vi "Initialize - Set Time Stamp.vi"(8 "error in (no error)":errorcluster, 11 "Device Item Ref in":T1 format="%.0x") -> (0 "error out":errorcluster, 2 "Path":string, 3 "Device Item Ref out":T1 format="%.0x")   [LabVIEW 2019, in "UDP-Custom-Device System Explorer.lvlib"]
doc: "Set the TimeStamp Ref Device Property to the System Time channel."
uses:
  UDP-Custom-Device System Explorer.lvlib
  <vilib>/NI VeriStand/Custom Device API/Custom Device Item Ref.ctl
  <vilib>/NI VeriStand/Custom Device Tools/Custom Device Utility Library/Custom Device Utility Library.lvlib
  <vilib>/NI VeriStand/Custom Device API/Custom Device API.lvlib
  Property Accessors/Main Accessors.lvlib
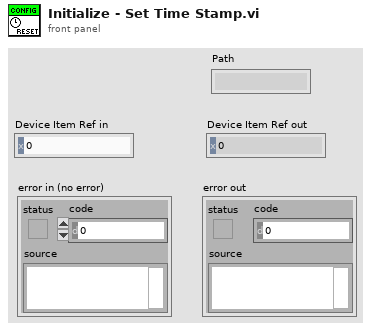
[diagram p1: front panel]
types:
  T1 = typedef "Custom Device API.lvlib/Custom Device Item Ref.ctl" = u64
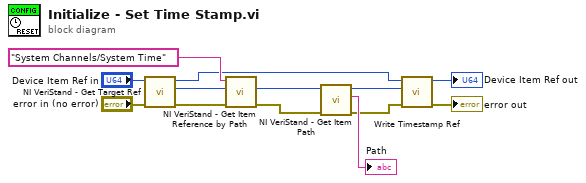
[diagram p0: block diagram]
diagram:
  n1 = call <vilib>:"NI VeriStand - Get Target Ref.vi"("error in"="error in (no error)", "Item Ref in"="Device Item Ref in") -> ("error out"=w12:errorcluster, "Target Ref"=w13:T1, "Item Ref out"=w5:T1)  [unwired: 6 in, 1 out]
  n2 = call <vilib>:"NI VeriStand - Get Item Reference by Path.vi"("error in (no error)"=w12, "Root Ref"=w13, "Item Path in"="System Channels/System Time" ("Relative Item Path")) -> ("error out"=w7:errorcluster, "Item Ref"=w8:T1)  [unwired: 5 in, 2 out]
  n3 = call <vilib>:"NI VeriStand - Get Item Path.vi"("error in (no error)"=w7, "Item Ref in"=w8) -> ("error out"=w4:errorcluster, "Path"=→"Path":string, "Item Ref out"=w2:T1)  [unwired: 6 in, 1 out]
  n4 = call "Write Timestamp Ref.vi"("error in (no error)"=w4, "Timestamp Ref"=w2, "Node Ptr"=w5) -> ("error out"=→"error out":errorcluster, "Node Ptr out"=→"Device Item Ref out":T1)  [unwired: 7 in]
